vi "Front Panel.vi"(11 "GUI In":refnum<class "PAS Housekeeping.lvclass">) -> ()   [LabVIEW 2015, in "PAS Housekeeping.lvclass"]
uses:
  PAS Housekeeping.lvclass
  Reusable/Xctls/Buffer/2D Control/2D Buffer Display.xctl
  Reusable/GUI/GUI.lvclass/GUI.ctl
  Reusable/Observer/Observer.lvclass/Observer.ctl
  Data/cPAS Data.lvclass
  Data/cPAS Cell Data/cPAS Cell Data.lvclass
  Data/cPAS Data.lvclass/cPAS Data.ctl
  Data/Read Serial Data.vi
  Reusable/GUI/Accessors/Read RegEvent.vi
  Reusable/Observer/Read Data Queue.vi
  Reusable/PAS/Data/Main/Read CellData.vi
  Data/Read Thum.vi
  Reusable/Data/Read measTime.vi
  Reusable/PAS/Data/Cell/Read houseKeeping.vi
  Data/Read T2_cell.vi
  Reusable/Data/Data.lvclass
  Reusable/PAS/Data/Cell/PAS Cell Data.lvclass
panel:
  out "pasHK":cluster{"data_out":sgl[][], "time":timestamp}(xcontrol)
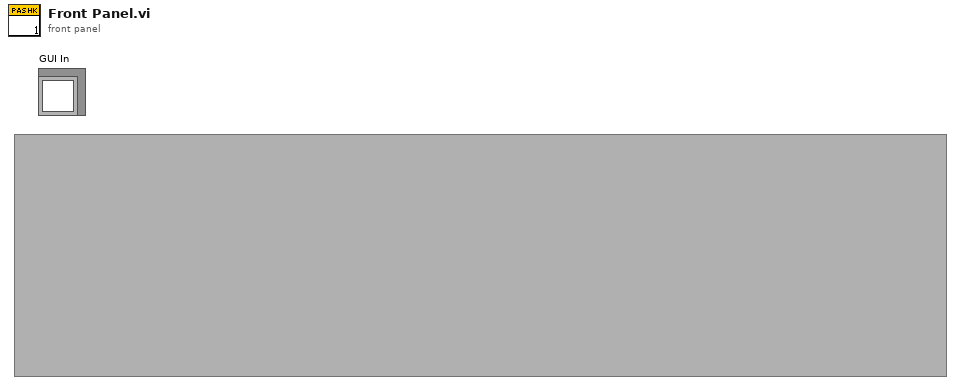
[diagram p1: front panel]
types:
  T1 = cluster{"Name":string, "Line Width":u8, "Line Style":u8, "Color":u32}[]
  T2 = cluster{"[0]":cluster{"Q":sgl, "T":sgl, "P":sgl}, "[1]":cluster{"Q":sgl, "T":sgl, "P":sgl}, "[2]":cluster{"Q":sgl, "T":sgl, "P":sgl}, "[3]":cluster{"Q":sgl, "T":sgl, "P":sgl}, "[4]":cluster{"Q":sgl, "T":sgl, "P":sgl}}
  T3 = cluster{"T":sgl, "TRH":sgl, "RH":sgl, "laserRMS":sgl}
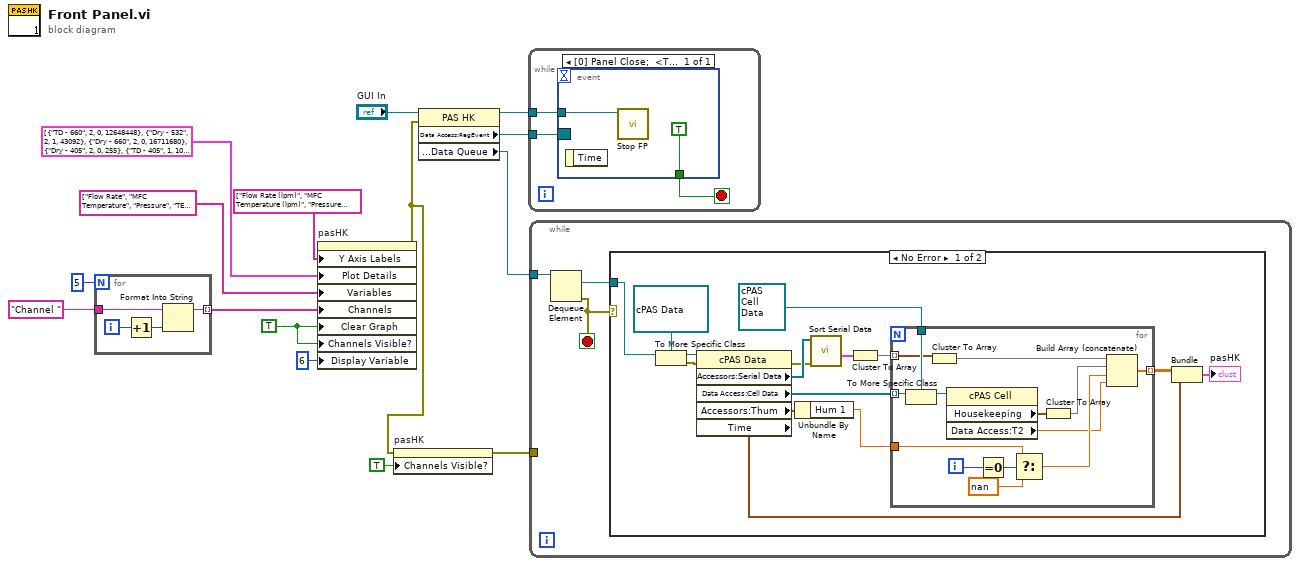
[diagram p0: block diagram]
diagram:
  w6 = TRUE ("Clear Graph")
  n1 = for {
    N: 5 -> [_]
    tunnel: "Channel " -> [w17]
    tunnel: [w16] -> w9 mode=indexing
    i -> [w19]
    n2 = Increment(x=w19) -> (x+1=w18:i32)
    n3 = Format Into String(initial string=w17, w18) -> (resulting string=w16:string)  [unwired: 2 in, 1 out]
  }
  n4 = property on="pasHK" class="2D Buffer Display (strict)"("Y Axis Labels"=string[] ["Flow Rate (lpm)", "MFC Temperature (lpm)", "Pressure (mb)", "TEC Thermistor Temperature (degC)", "Vaisala Temperature (degC)", "Relative Humidity (%)", "Laser RMS", "Saturator Temperature (degC)", "Thermistor "], "Plot Details"=T1 [{"Name"="TD - 660", "Line Width"=2, "Line Style"=0, "Color"=12648448}, {"Name"="Dry - 532", "Line Width"=2, "Line Style"=1, "Color"=43092}, {"Name"="Dry - 660", "Line Width"=2, "Line Style"=0, "Color"=16711680}, {"Name"="Dry - 405", "Line Width"=2, "Line Style"=0, "Color"=255}, {"Name"="TD - 405", "Line Width"=1, "Line Style"=10, "Color"=128}], "Variables"=string[] ["Flow Rate", "MFC Temperature", "Pressure", "TEC Thermistor Temperature", "Vaisala Temperature", "Relative Humidity", "Laser RMS", "Saturator Temperature", "Thermistor Temperature"], "Channels"=w9, "Clear Graph"=w6, "Channels Visible?"=w6, "Display Variable"=6) -> (error out=w3:errorcluster)  [unwired: 2 in, 1 out]
  n5 = property on="pasHK" class="2D Buffer Display (strict)"(error in=w3, "Channels Visible?"=TRUE) -> (error out=w2:errorcluster)  [unwired: 1 in, 1 out]
  n6 = property class="PAS HK"(reference="GUI In", error in=w3) -> (reference out=w7:refnum<class "PAS Housekeeping.lvclass">, "Data Access:RegEvent"=w15:refnum<event-registration>, "Data Access:Data Queue"=w14:refnum<queue>)  [unwired: 1 out]
  n7 = while {
    tunnel: w15 -> [w21]
    tunnel: w7 -> [w20]
    stop <- w22 stop-if-true
    n8 = event shown="[0] Panel Close;  <True>: User Event" {
      selector: w21 -> [_]
      dyn-events: _ -> [_]
      timeout: _ -> [_]
      tunnel: [TRUE] -> w22
      tunnel: w20 -> [w23]
      event Panel Close; User Event {
        n9 = event-data() -> ()  [unwired: 1 in, 1 out]
        n10 = call-dynamic "Stop FP.vi"("GUI in"=w23) -> ()  [unwired: 9 in, 2 out]
      }
    }
  }
  n11 = while {
    tunnel: w14 -> [w27]
    tunnel: w2 -> [_]
    stop <- w26 stop-if-true
    n12 = Dequeue Element(queue=w27) -> (element=w25:refnum<data-value>, error out=w26:errorcluster)  [unwired: 2 in, 2 out]
    n13 = case shown="No Error" w26 {
      tunnel: w25 -> [w42 _]
      frame No Error {
        n14 = To More Specific Class(target class=refnum<data-value> refnum ("data value reference"), reference=w42) -> (specific class reference=w40:refnum<data-value>, error out=w39:errorcluster)  [unwired: 1 in]
        n15 = property class="cPAS Data"(reference=w40, error in=w39) -> (error out=w34:errorcluster, "Accessors:Serial Data"=w35:refnum<class "Data.lvclass">[], "Data Access:Cell Data"=w36:refnum<class "PAS Cell Data.lvclass">[], "Accessors:Thum"=w30:cluster{"Hum 1":sgl, "Hum 2":sgl}, "Time"=w31:timestamp)  [unwired: 1 out]
        n16 = Unbundle By Name(w30) -> ("Hum 1"=w29:sgl)
        n17 = call "Sort Serial Data.vi"("error in"=w34, "SerialData"=w35) -> ("acatDataOut"=w33:T2)  [unwired: 7 in, 2 out]
        n18 = Cluster To Array(cluster=w33) -> (array=w32:cluster{"Q":sgl, "T":sgl, "P":sgl}[])
        n19 = for {
          tunnel: w36 -> [w56] mode=indexing
          tunnel: [w43] -> w38 mode=indexing
          tunnel: refnum<class "cPAS Cell Data.lvclass"> refnum ("cPAS Cell") -> [w54]
          tunnel: w32 -> [w51] mode=indexing
          tunnel: w29 -> [w47]
          i -> [w49]
          n20 = To More Specific Class(target class=w54, reference=w56) -> (specific class reference=w55:refnum<class "cPAS Cell Data.lvclass">)  [unwired: 1 in, 1 out]
          n21 = Cluster To Array(cluster=w51) -> (array=w50:sgl[])
          n22 = property class="cPAS Cell"(reference=w55) -> ("Housekeeping"=w53:T3, "Data Access:T2"=w44:sgl)  [unwired: 1 in, 2 out]
          n23 = Equal To 0?(x=w49) -> (x = 0?=w48:bool)
          n24 = Select(t=w47, s=w48, f=sgl nan) -> (s? t:f=w45:sgl)
          n25 = Cluster To Array(cluster=w53) -> (array=w52:sgl[])
          n26 = Build Array (concatenate)(w50, w52, w45, w44) -> (w43:sgl[])
        }
        n27 = Bundle(w38, "Time"=w31) -> (→"pasHK":cluster{sgl[][], "Time":timestamp})  [unwired: 1 in]
      }
      frame Error {
      }
    }
  }
